vi "ClearSpecificError.vi"(8 "error in":errorcluster, 11 "code":i32) -> (0 "error out":errorcluster, 2 "error cleared?":bool)   [LabVIEW 2023, in "CEF.lvlib"]
doc: "Clears the Error if it matches the specific codeCopyright 2017 National Instruments Corporation\n\nLicensed under the Apache License, Version 2.0 (the \"License\"); you may not use this file except in compliance with the License. You may obtain a copy of the License at http://www.apache.org/licenses/LICENSE-2.0\nUnless required by applicable law or agreed to in writing, software distributed under the License is distributed on an \"AS IS\" BASIS, WITHOUT WARRANTIES OR CONDITIONS OF ANY KIND, either express or implied. See the License for the specific language governing permissions and limitations under the License."
uses:
  CEF.lvlib
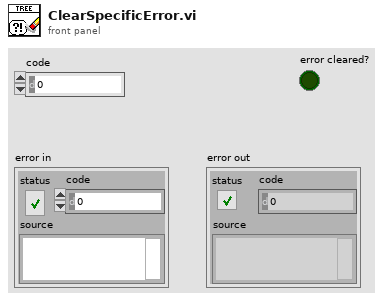
[diagram p1: front panel]
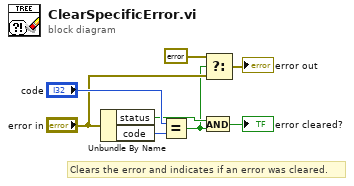
[diagram p0: block diagram]
diagram:
  # "Clears the error and indicates if an error was cleared."
  n1 = Unbundle By Name("error in") -> ("status"=w3:bool, "code"=w7:i32)
  n2 = Equal?(x="code", y=w7) -> (x = y?=w2:bool)
  n3 = And(x=w3, y=w2) -> (x .and. y?=→"error cleared?":bool)
  n4 = Select(t=errorcluster {"status"=FALSE, "code"=0, "source"=""}, s=w2, f="error in") -> (s? t:f=→"error out":errorcluster)
